vi "treeTraversComponentsRecursive.vi"(7 "Cluster in":T2, 8 "error in (no error)":errorcluster, 9 "DisplayType":T1=enum."UNSPECIFIED", 10 "Component":refnum<class "IComponent.lvclass">) -> (0 "error out":errorcluster, 5 "Cluster out":T2)   [LabVIEW 2022 SP3, in "Property Editor.lvlib"]
uses:
  Property Editor.lvlib
  Public/Classes/IComponent/IComponent.lvclass
  Public/Classes/IBaseObject/IBaseObject.lvclass
  Public/Classes/IFolder/IFolder.lvclass
  Public/Classes/IDevice/IDevice.lvclass
  TypeDef/DisplayType.ctl
  Public/Classes/IBaseObject/Polymorphic/borrowInterface/borrowSignalInterface.vi
  Public/Classes/IBaseObject/Polymorphic/borrowInterface/borrowChannelInterface.vi
  Public/Classes/IBaseObject/Polymorphic/borrowInterface/borrowFunctionBlockInterface.vi
  Public/Classes/IBaseObject/Polymorphic/borrowInterface/borrowFolderInterface.vi
  Public/Classes/IBaseObject/Polymorphic/borrowInterface/borrowServerInterface.vi
  Public/Classes/IBaseObject/Polymorphic/borrowInterface/borrowInputPortInterface.vi
  Public/Classes/IBaseObject/Polymorphic/borrowInterface/borrowDeviceInterface.vi
  TypeDef/Context.ctl
  Public/Classes/IProperty/IProperty.lvclass
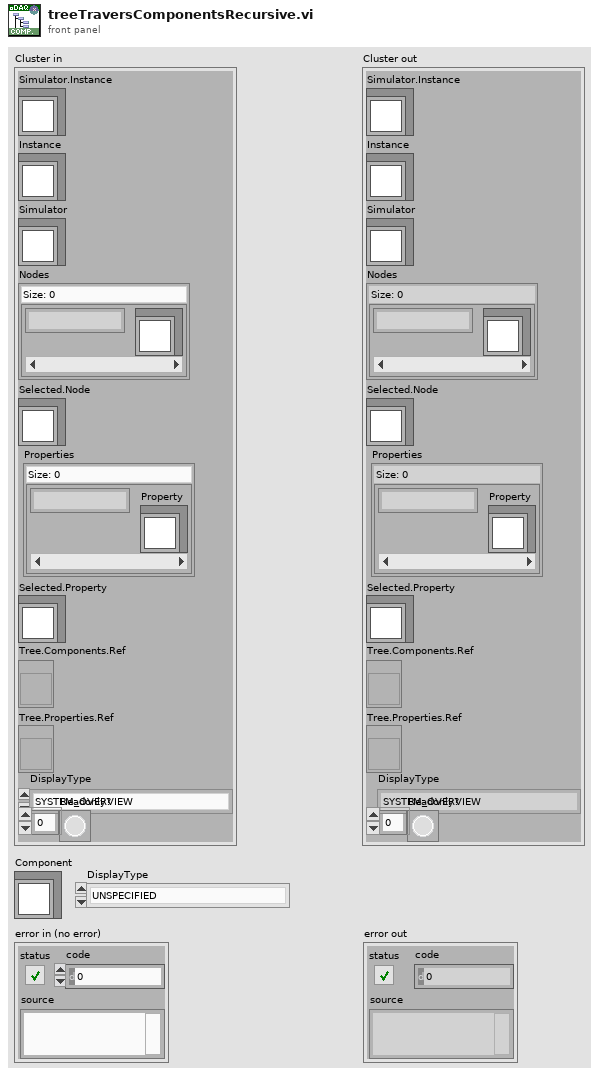
[diagram p1: front panel]
types:
  T1 = typedef "Property Editor.lvlib/DisplayType.ctl" = enum16{"SYSTEM_OVERVIEW", "SIGNALS", "CHANNELS", "FUNCTION_BLOCKS", "TOPOLOGY", "TOPOLOGY_CUSTOM_COMPONENTS", "UNSPECIFIED"}
  T2 = typedef "Property Editor.lvlib/Context.ctl" = cluster{"Simulator.Instance":refnum<class "IComponent.lvclass">, "Instance":refnum<class "IComponent.lvclass">, "Simulator":refnum<class "IComponent.lvclass">, "Nodes":map{string, refnum<class "IComponent.lvclass">}, "Selected.Node":refnum<class "IComponent.lvclass">, "Properties":map{string, refnum<class "IProperty.lvclass">}, "Selected.Property":refnum<class "IProperty.lvclass">, "Tree.Components.Ref":refnum<vi>, "Tree.Properties.Ref":refnum<vi>, "DisplayType":T1, "Readonly?":bool[]}
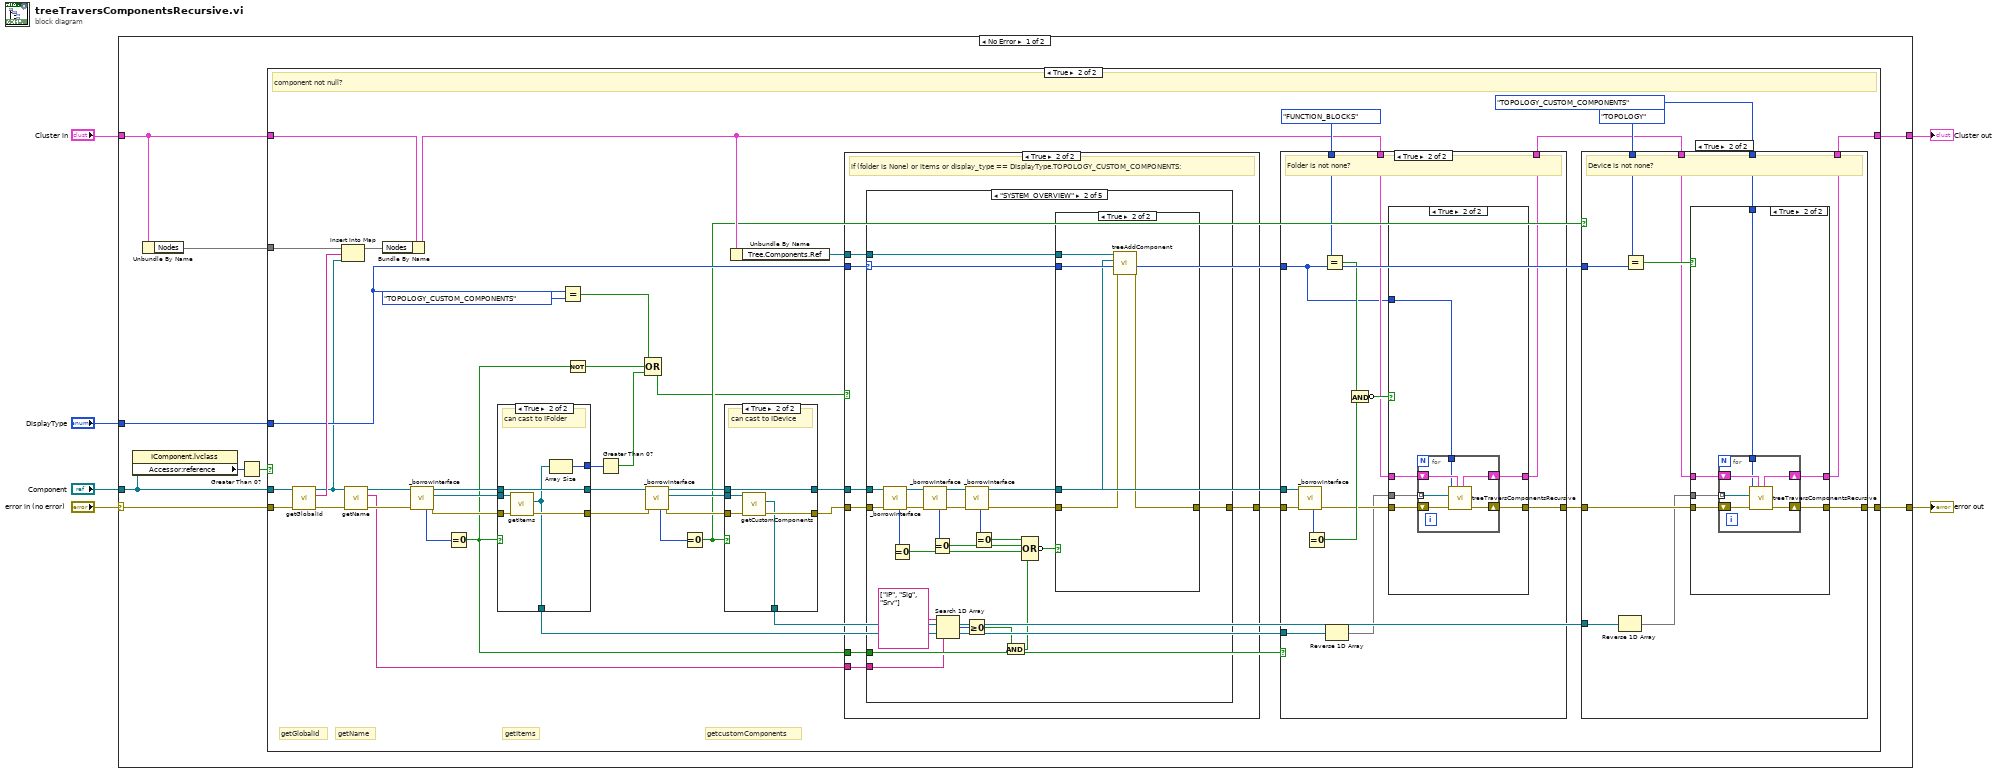
[diagram p0: block diagram]
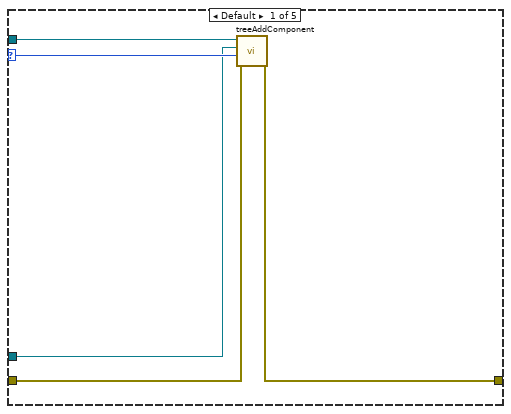
[diagram p9: hidden frame]
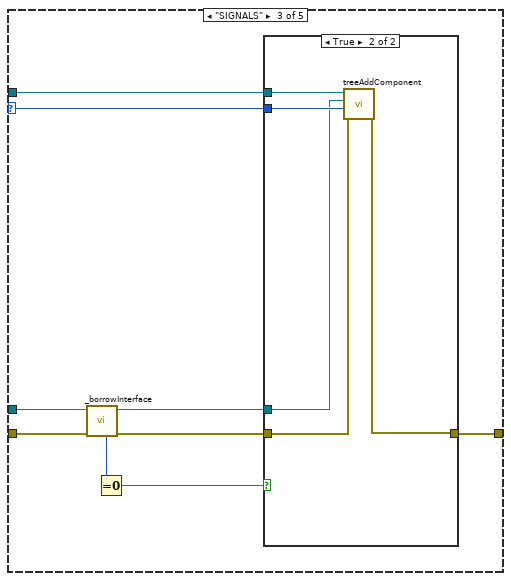
[diagram p11: hidden frame]
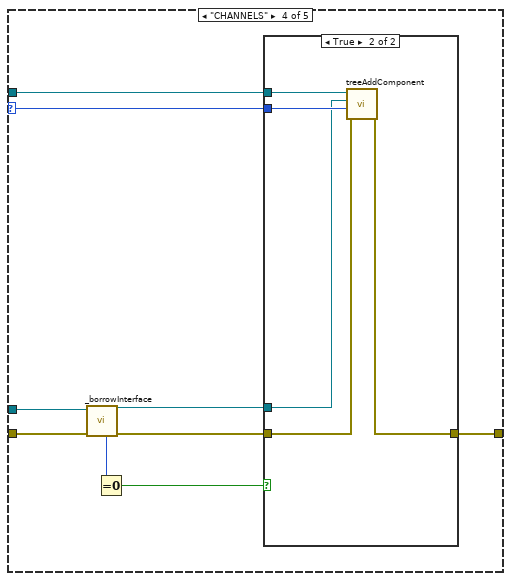
[diagram p13: hidden frame]
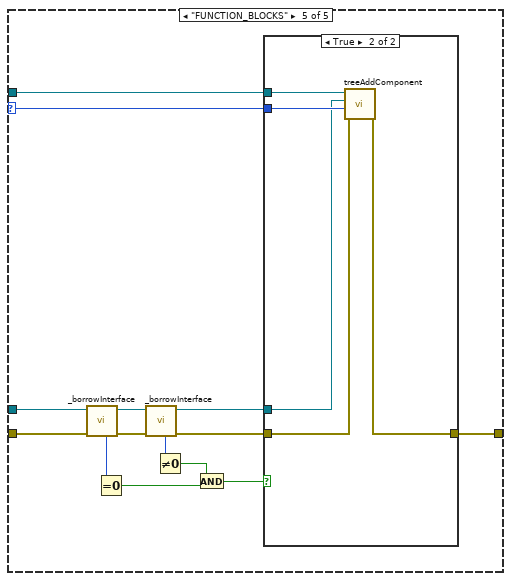
[diagram p15: hidden frame]
diagram:
  n1 = case shown="No Error" "error in (no error)" {
    selector: "error in (no error)" -> [w14 w226]
    tunnel: [w13 w227] -> w6
    tunnel: "Cluster in" -> [w15 w227]
    tunnel: [w12 w226] -> w4
    tunnel: "Component" -> [w10 _]
    tunnel: "DisplayType" -> [w7 _]
    frame No Error {
      n2 = property class="IComponent.lvclass"(reference=w10) -> ("Accessor:reference"=w11:i64)  [unwired: 1 in, 2 out]
      n3 = Unbundle By Name(w15) -> ("Nodes"=w8:map{string, refnum<class "IComponent.lvclass">})
      n4 = Greater Than 0?(x=w11) -> (x > 0?=w9:bool)
      n5 = case shown="True" w9 {
        tunnel: w15 -> [w17 w54]
        tunnel: w14 -> [w16 w53]
        tunnel: w10 -> [_ w44]
        tunnel: [w17 w29] -> w13
        tunnel: [w16 w27] -> w12
        tunnel: w8 -> [_ w38]
        tunnel: w7 -> [_ w26]
        frame False {
          # "component not null?"
        }
        frame True {
          # "getcustomComponents"
          # "getItems"
          # "getName"
          # "getGlobalId"
          # "component not null?"
          n6 = call "getGlobalId.vi"("error in (no error)"=w53, "IComponent in"=w44) -> ("error out"=w19:errorcluster, "GlobalId out"=w57:string, "IComponent out"=w18:refnum<class "IComponent.lvclass">)  [unwired: 7 in]
          n7 = Insert Into Map(map in=w38, key=w57, value=w18) -> (map out=w55:map{string, refnum<class "IComponent.lvclass">})  [unwired: 2 out]
          n8 = call "getName.vi"("error in (no error)"=w19, "IComponent in"=w18) -> ("error out"=w42:errorcluster, "Name out"=w24:string, "IComponent out"=w43:refnum<class "IComponent.lvclass">)  [unwired: 7 in]
          n9 = Bundle By Name(cluster=w54, "Nodes"=w55) -> (w35:T2)
          n10 = call-poly "_borrowInterface.vi"("error in (no error)"=w42, "IBaseObject in"=w43) -> ("error out"=w51:errorcluster, "Folder out"=w41:refnum<class "IFolder.lvclass">, "IBaseObject out"=w50:refnum<class "IComponent.lvclass">, "err"=w52:u32)  [unwired: 6 in]
          n11 = Equal To 0?(x=w52) -> (x = 0?=w22:bool)
          n12 = case shown="True" w22 {
            tunnel: [w119 w125] -> w46
            tunnel: w51 -> [w119 w124]
            tunnel: w41 -> [_ w123]
            tunnel: w50 -> [w118 w122]
            tunnel: [w118 w122] -> w45
            tunnel: [_ w121] -> w40
            tunnel: [_ w120] -> w34
            frame False {
            }
            frame True {
              # "can cast to IFolder"
              n13 = call "getItems.vi"("error in (no error)"=w124, "IFolder in"=w123) -> ("error out"=w125:errorcluster, "Components out"=w120:refnum<class "IComponent.lvclass">[])  [unwired: 7 in, 1 out]
              n14 = Array Size(array=w120) -> (size(s)=w121:i32)
            }
          }
          n15 = Equal?(x=w26, y=DisplayType."TOPOLOGY_CUSTOM_COMPONENTS") -> (x = y?=w59:bool)
          n16 = Not(x=w22) -> (.not. x?=w21:bool)
          n17 = Greater Than 0?(x=w40) -> (x > 0?=w58:bool)
          n18 = Compound Arithmetic op=OR(w59, w21, w58) -> (w20:bool)
          n19 = call-poly "_borrowInterface.vi"("error in (no error)"=w46, "IBaseObject in"=w45) -> ("error out"=w48:errorcluster, "Device out"=w32:refnum<class "IDevice.lvclass">, "IBaseObject out"=w49:refnum<class "IComponent.lvclass">, "err"=w47:u32)  [unwired: 6 in]
          n20 = Equal To 0?(x=w47) -> (x = 0?=w23:bool)
          n21 = case shown="True" w23 {
            tunnel: [w220 w222] -> w37
            tunnel: w48 -> [w220 w223]
            tunnel: w32 -> [_ w224]
            tunnel: w49 -> [w219 w225]
            tunnel: [w219 w225] -> w33
            tunnel: [_ w221] -> w28
            frame False {
            }
            frame True {
              # "can cast to IDevice"
              n22 = call "getCustomComponents.vi"("error in (no error)"=w223, "IDevice in"=w224) -> ("error out"=w222:errorcluster, "CustomComponents out"=w221:refnum<class "IComponent.lvclass">[])  [unwired: 7 in, 1 out]
            }
          }
          n23 = Unbundle By Name(w35) -> ("Tree.Components.Ref"=w56:refnum<vi>)
          n24 = case shown="True" w20 {
            tunnel: w56 -> [_ w133]
            tunnel: [w126 w132] -> w36
            tunnel: w22 -> [_ w128]
            tunnel: w33 -> [_ w131]
            tunnel: w37 -> [w126 w130]
            tunnel: w24 -> [_ w129]
            tunnel: w26 -> [_ w127]
            frame False {
            }
            frame True {
              # "if (folder is None) or items or display_type == DisplayType.TOPOLOGY_CUSTOM_COMPONENTS:"
              n25 = case shown="\"SYSTEM_OVERVIEW\"" w127 {
                selector: w127 -> [w137 w140 w170 w185 w200]
                tunnel: w133 -> [w138 w141 w177 w192 w201]
                tunnel: [w135 w162 w176 w191 w212] -> w132
                tunnel: w131 -> [w134 w161 w174 w189 w210]
                tunnel: w130 -> [w136 w160 w173 w188 w209]
                tunnel: w129 -> [_ w145 _ _ _]
                tunnel: w128 -> [_ w144 _ _ _]
                frame Default {
                  n26 = call "treeAddComponent.vi"("error in (no error)"=w136, "DisplayType in"=w137, "Component in"=w134, "Tree Ref in"=w138) -> ("error out"=w135:errorcluster)  [unwired: 6 in, 1 out]
                }
                frame "SYSTEM_OVERVIEW" {
                  n27 = call-poly "_borrowInterface.vi"("error in (no error)"=w160, "IBaseObject in"=w161) -> ("error out"=w158:errorcluster, "IBaseObject out"=w159:refnum<class "IComponent.lvclass">, "err"=w155:u32)  [unwired: 6 in, 1 out]
                  n28 = Equal To 0?(x=w155) -> (x = 0?=w150:bool)
                  n29 = call-poly "_borrowInterface.vi"("error in (no error)"=w158, "IBaseObject in"=w159) -> ("error out"=w156:errorcluster, "IBaseObject out"=w157:refnum<class "IComponent.lvclass">, "err"=w154:u32)  [unwired: 6 in, 1 out]
                  n30 = Equal To 0?(x=w154) -> (x = 0?=w151:bool)
                  n31 = Search 1D Array(1D array=string[] ["IP", "Sig", "Srv"], element=w145) -> (index of element=w143:i32)  [unwired: 1 in]
                  n32 = call-poly "_borrowInterface.vi"("error in (no error)"=w156, "IBaseObject in"=w157) -> ("error out"=w149:errorcluster, "IBaseObject out"=w139:refnum<class "IComponent.lvclass">, "err"=w153:u32)  [unwired: 6 in, 1 out]
                  n33 = Greater Or Equal To 0?(x=w143) -> (x >= 0?=w142:bool)
                  n34 = Equal To 0?(x=w153) -> (x = 0?=w152:bool)
                  n35 = And(x=w142, y=w144) -> (x .and. y?=w148:bool)
                  n36 = Compound Arithmetic op=OR(w152, w151, w150, w148) -> (invert w147:bool)
                  n37 = case shown="True" w147 {
                    tunnel: [w163 w166] -> w162
                    tunnel: w149 -> [w163 w167]
                    tunnel: w141 -> [_ w168]
                    tunnel: w140 -> [_ w165]
                    tunnel: w139 -> [_ w164]
                    frame False {
                    }
                    frame True {
                      n38 = call "treeAddComponent.vi"("error in (no error)"=w167, "DisplayType in"=w165, "Component in"=w164, "Tree Ref in"=w168) -> ("error out"=w166:errorcluster)  [unwired: 6 in, 1 out]
                    }
                  }
                }
                frame "SIGNALS" {
                  n39 = call-poly "_borrowInterface.vi"("error in (no error)"=w173, "IBaseObject in"=w174) -> ("error out"=w171:errorcluster, "IBaseObject out"=w169:refnum<class "IComponent.lvclass">, "err"=w175:u32)  [unwired: 6 in, 1 out]
                  n40 = Equal To 0?(x=w175) -> (x = 0?=w172:bool)
                  n41 = case shown="True" w172 {
                    tunnel: w177 -> [_ w183]
                    tunnel: [w178 w180] -> w176
                    tunnel: w171 -> [w178 w181]
                    tunnel: w170 -> [_ w182]
                    tunnel: w169 -> [_ w179]
                    frame False {
                    }
                    frame True {
                      n42 = call "treeAddComponent.vi"("error in (no error)"=w181, "DisplayType in"=w182, "Component in"=w179, "Tree Ref in"=w183) -> ("error out"=w180:errorcluster)  [unwired: 6 in, 1 out]
                    }
                  }
                }
                frame "CHANNELS" {
                  n43 = call-poly "_borrowInterface.vi"("error in (no error)"=w188, "IBaseObject in"=w189) -> ("error out"=w186:errorcluster, "IBaseObject out"=w184:refnum<class "IComponent.lvclass">, "err"=w190:u32)  [unwired: 6 in, 1 out]
                  n44 = Equal To 0?(x=w190) -> (x = 0?=w187:bool)
                  n45 = case shown="True" w187 {
                    tunnel: w192 -> [_ w198]
                    tunnel: [w193 w195] -> w191
                    tunnel: w186 -> [w193 w196]
                    tunnel: w185 -> [_ w197]
                    tunnel: w184 -> [_ w194]
                    frame False {
                    }
                    frame True {
                      n46 = call "treeAddComponent.vi"("error in (no error)"=w196, "DisplayType in"=w197, "Component in"=w194, "Tree Ref in"=w198) -> ("error out"=w195:errorcluster)  [unwired: 6 in, 1 out]
                    }
                  }
                }
                frame "FUNCTION_BLOCKS" {
                  n47 = call-poly "_borrowInterface.vi"("error in (no error)"=w209, "IBaseObject in"=w210) -> ("error out"=w207:errorcluster, "IBaseObject out"=w208:refnum<class "IComponent.lvclass">, "err"=w211:u32)  [unwired: 6 in, 1 out]
                  n48 = Equal To 0?(x=w211) -> (x = 0?=w202:bool)
                  n49 = call-poly "_borrowInterface.vi"("error in (no error)"=w207, "IBaseObject in"=w208) -> ("error out"=w206:errorcluster, "IBaseObject out"=w199:refnum<class "IComponent.lvclass">, "err"=w205:u32)  [unwired: 6 in, 1 out]
                  n50 = Not Equal To 0?(x=w205) -> (x != 0?=w204:bool)
                  n51 = And(x=w204, y=w202) -> (x .and. y?=w203:bool)
                  n52 = case shown="True" w203 {
                    tunnel: [w213 w216] -> w212
                    tunnel: w206 -> [w213 w217]
                    tunnel: w201 -> [_ w218]
                    tunnel: w200 -> [_ w215]
                    tunnel: w199 -> [_ w214]
                    frame False {
                    }
                    frame True {
                      n53 = call "treeAddComponent.vi"("error in (no error)"=w217, "DisplayType in"=w215, "Component in"=w214, "Tree Ref in"=w218) -> ("error out"=w216:errorcluster)  [unwired: 6 in, 1 out]
                    }
                  }
                }
              }
            }
          }
          n54 = case shown="True" w22 {
            tunnel: w36 -> [w89 w102]
            tunnel: [w89 w98] -> w31
            tunnel: w26 -> [_ w90]
            tunnel: DisplayType."FUNCTION_BLOCKS" ("y") -> [_ w97]
            tunnel: w35 -> [w88 w95]
            tunnel: [w88 w94] -> w30
            tunnel: w34 -> [_ w93]
            tunnel: w33 -> [_ w92]
            frame False {
              # "Folder is not none?"
            }
            frame True {
              # "Folder is not none?"
              n55 = call-poly "_borrowInterface.vi"("error in (no error)"=w102, "IBaseObject in"=w92) -> ("error out"=w99:errorcluster, "err"=w103:u32)  [unwired: 6 in, 2 out]
              n56 = Equal To 0?(x=w103) -> (x = 0?=w100:bool)
              n57 = Equal?(x=w97, y=w90) -> (x = y?=w101:bool)
              n58 = Reverse 1D Array(array=w93) -> (reversed array=w91:refnum<class "IComponent.lvclass">[])
              n59 = Compound Arithmetic op=AND(w101, w100) -> (invert w96:bool)
              n60 = case shown="True" w96 {
                tunnel: w99 -> [w105 w111]
                tunnel: [w105 w110] -> w98
                tunnel: w95 -> [w104 w109]
                tunnel: [w104 w107] -> w94
                tunnel: w91 -> [_ w108]
                tunnel: w90 -> [_ w106]
                frame False {
                }
                frame True {
                  n61 = for {
                    shift-right: [w116] -> w110
                    shift-left: w111 -> [w117]
                    tunnel: w108 -> [w113] mode=indexing
                    shift-right: [w114] -> w107
                    shift-left: w109 -> [w115]
                    tunnel: w106 -> [w112]
                    n62 = call "treeTraversComponentsRecursive.vi"("Cluster in"=w115, "error in (no error)"=w117, "DisplayType"=w112, "Component"=w113) -> ("error out"=w116:errorcluster, "Cluster out"=w114:T2)  [unwired: 6 in]
                  }
                }
              }
            }
          }
          n63 = case shown="True" w23 {
            tunnel: w31 -> [w63 w66]
            tunnel: [w63 w72] -> w27
            tunnel: w26 -> [_ w71]
            tunnel: DisplayType."TOPOLOGY" ("y") -> [_ w70]
            tunnel: w30 -> [w62 w69]
            tunnel: [w62 w68] -> w29
            tunnel: w28 -> [_ w67]
            tunnel: DisplayType."TOPOLOGY_CUSTOM_COMPONENTS" ("y") -> [_ w65]
            frame False {
              # "Folder is not none?"
            }
            frame True {
              # "Device is not none?"
              n64 = Reverse 1D Array(array=w67) -> (reversed array=w64:refnum<class "IComponent.lvclass">[])
              n65 = Equal?(x=w70, y=w71) -> (x = y?=w73:bool)
              n66 = case shown="True" w73 {
                tunnel: w66 -> [w75 w81]
                tunnel: [w75 w80] -> w72
                tunnel: w69 -> [w74 w79]
                tunnel: [w74 w77] -> w68
                tunnel: w64 -> [_ w78]
                tunnel: w65 -> [_ w76]
                frame False {
                }
                frame True {
                  n67 = for {
                    shift-right: [w86] -> w80
                    shift-left: w81 -> [w87]
                    tunnel: w78 -> [w83] mode=indexing
                    shift-right: [w84] -> w77
                    shift-left: w79 -> [w85]
                    tunnel: w76 -> [w82]
                    n68 = call "treeTraversComponentsRecursive.vi"("Cluster in"=w85, "error in (no error)"=w87, "DisplayType"=w82, "Component"=w83) -> ("error out"=w86:errorcluster, "Cluster out"=w84:T2)  [unwired: 6 in]
                  }
                }
              }
            }
          }
        }
      }
    }
    frame Error {
    }
  }
  "Cluster out" <- w6
  "error out" <- w4
